vi "Lex Text-{} UnescapedVariable.vi"(8 "Error In":errorcluster) -> (0 "Error Out":errorcluster)   [LabVIEW 2018, in "Tests.lvlib" / "Lexer.lvlib"]
uses:
  Lexer.lvlib
  src/Toolkit/Low-Level/Tokens/Text/Text.lvclass
  src/Toolkit/Low-Level/Tokens/UnescapedVariable/UnescapedVariable.lvclass
  <vilib>/addons/_JKI Toolkits/Caraya/classes/Assert/Assert Equal Type_Variant.vi
  src/Toolkit/Low-Level/Tokens/Contentable/Contentable.lvclass
  src/Toolkit/Low-Level/Tokens/Keyable/Keyable.lvclass
  src/Toolkit/Low-Level/Lexer/Lexer.lvclass
  <vilib>/addons/_JKI Toolkits/Caraya/classes/Test/Test.lvclass
  <vilib>/addons/_JKI Toolkits/Caraya/classes/Assert/Assert.lvclass
  src/Toolkit/Low-Level/Tokens/Token/Token.lvclass
  Tests.lvlib
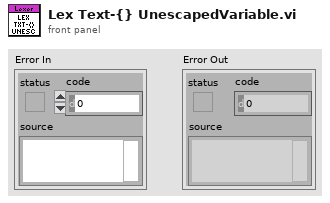
[diagram p1: front panel]
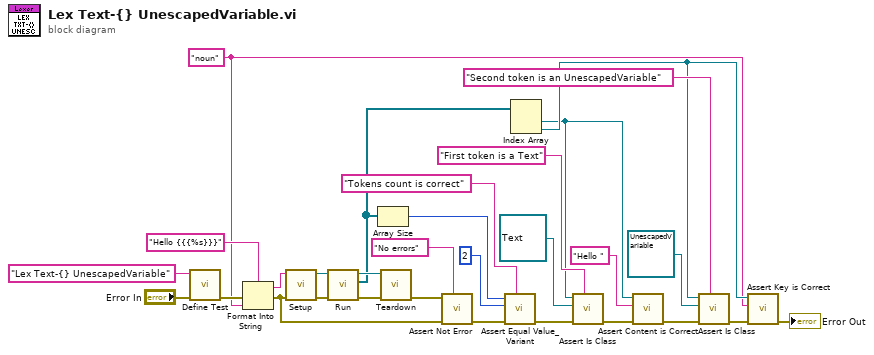
[diagram p0: block diagram]
diagram:
  w11 = "noun" ("String")
  n1 = call <vilib>:"Define Test.vi"("error in (no error)"="Error In", "Label (VI Title)"="Lex Text-{} UnescapedVariable") -> ("error out"=w28:errorcluster)  [unwired: 9 in]
  n2 = Format Into String(format string="Hello {{{%s}}}", error in=w28, w11) -> (resulting string=w3:string, error out=w4:errorcluster)  [unwired: 1 in]
  n3 = call "Setup.vi"("Error In"=w4, "String"=w3) -> ("Error Out"=w7:errorcluster, "Lexer"=w8:refnum<class "Lexer.lvclass">)  [unwired: 8 in]
  n4 = call-dynamic "Run.vi"("Error In"=w7, "Lexer In"=w8) -> ("Error Out"=w5:errorcluster, "Tokens"=w1:refnum<class "Token.lvclass">[], "Lexer Out"=w6:refnum<class "Lexer.lvclass">)  [unwired: 7 in]
  n5 = Array Size(array=w1) -> (size(s)=w24:i32)
  n6 = call "Teardown.vi"("Error In"=w5, "Lexer"=w6) -> ("Error Out"=w2:errorcluster)  [unwired: 9 in]
  n7 = call <vilib>:"Assert Not Error.vi"("Label"="No errors", "error in (no error)"=w4, "Not Error?"=w2) -> ("error out"=w26:errorcluster)  [unwired: 8 in]
  n8 = call <vilib>:"Assert Equal Value_Variant.vi"("Label"="Tokens count is correct", "error in (no error)"=w26, "Y"=2 ("size(s)"), "X"=w24) -> ("error out"=w22:errorcluster)  [unwired: 7 in]
  n9 = Index Array(array=w1) -> (element #1=w10:refnum<class "Token.lvclass">, element #2=w13:refnum<class "Token.lvclass">)  [unwired: 2 in]
  n10 = call "Assert Is Class.vi"("Label"="First token is a Text", "Error In"=w22, "Expected"=refnum<class "Text.lvclass"> refnum ("Mustache.lvlib:Tokens.lvlib:Text.lvclass"), "Actual"=w10) -> ("Error Out"=w20:errorcluster)  [unwired: 7 in]
  n11 = call "Assert Content is Correct.vi"("Error In"=w20, "Expected"="Hello ", "Token"=w10) -> ("Error Out"=w19:errorcluster)  [unwired: 8 in]
  n12 = call "Assert Is Class.vi"("Label"="Second token is an UnescapedVariable", "Error In"=w19, "Expected"=refnum<class "UnescapedVariable.lvclass"> refnum ("Mustache.lvlib:Tokens.lvlib:UnescapedVariable.lvclass"), "Actual"=w13) -> ("Error Out"=w12:errorcluster)  [unwired: 7 in]
  n13 = call "Assert Key is Correct.vi"("Error In"=w12, "Expected"=w11, "Token"=w13) -> ("Error Out"=→"Error Out":errorcluster)  [unwired: 8 in]
